vi "LB_AssertIndexValue_Tests.vi"(11 "error in":errorcluster) -> (15 "error out":errorcluster)   [LabVIEW 2016, in "DronaTest.lvlib"]
uses:
  DronaTest.lvlib
  APIs/Stimulus/ControlValue/SetValueAuto.vi
  APIs/Assert/AssertControlValue/Controls/Listbox/AssertIndexValue.vi
  <vilib>/addons/_JKI Toolkits/Caraya/classes/Assert/Assert Error.vi
  <vilib>/addons/_JKI Toolkits/Caraya/classes/Assert/Assert Equal Value_Variant.vi
  <vilib>/addons/_JKI Toolkits/Caraya/classes/Test/Test.lvclass
  Drona.lvlib
  <vilib>/SLL Toolkit/SLL Debug/SLL Debug.lvlib
  <vilib>/addons/_JKI Toolkits/Caraya/classes/Assert/Assert.lvclass
  APIs/Assert/AssertControlValue/Controls/Listbox/AssertListbox.lvlib
  APIs/Stimulus/ControlValue/ControlValue.lvlib
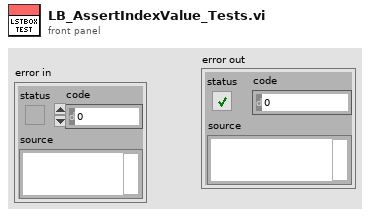
[diagram p1: front panel]
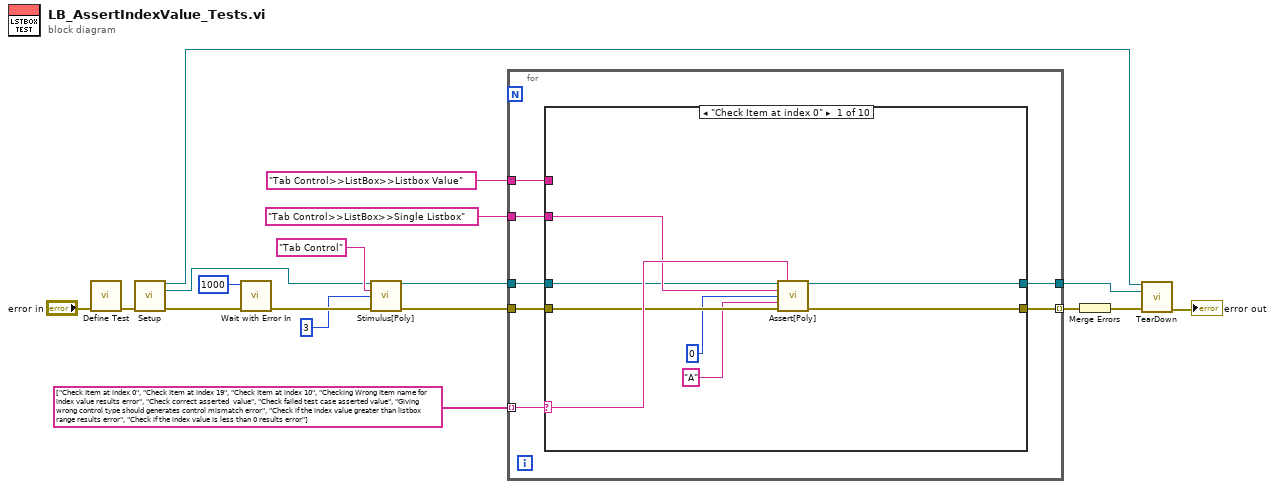
[diagram p0: block diagram]
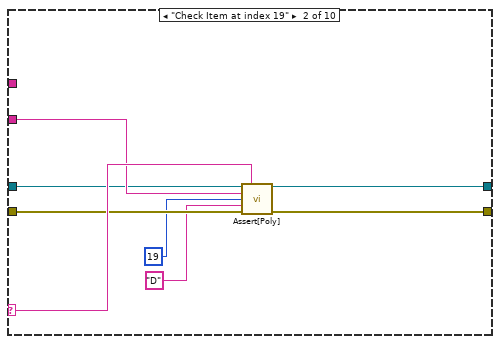
[diagram p2: hidden frame]
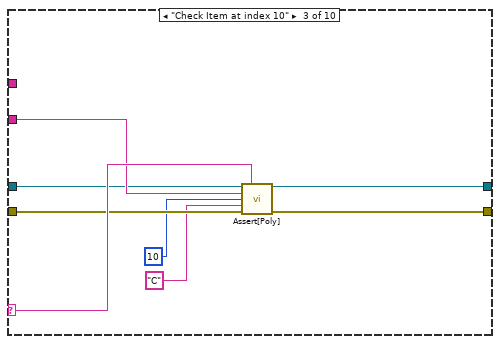
[diagram p3: hidden frame]
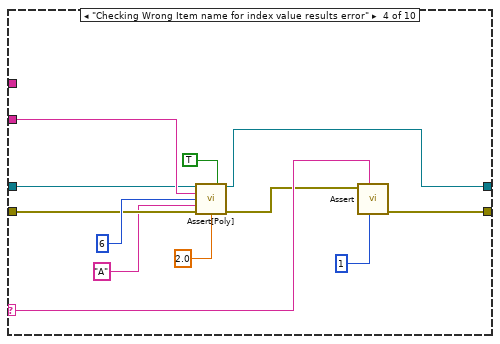
[diagram p4: hidden frame]
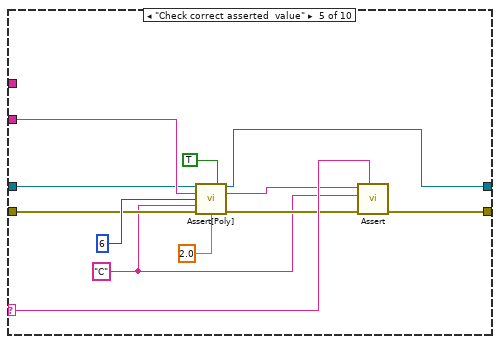
[diagram p5: hidden frame]
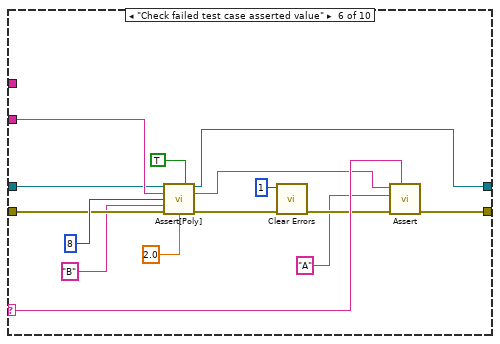
[diagram p6: hidden frame]
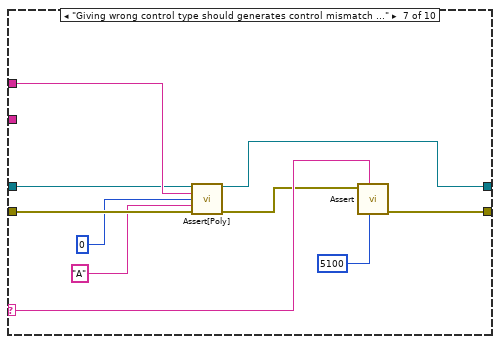
[diagram p7: hidden frame]
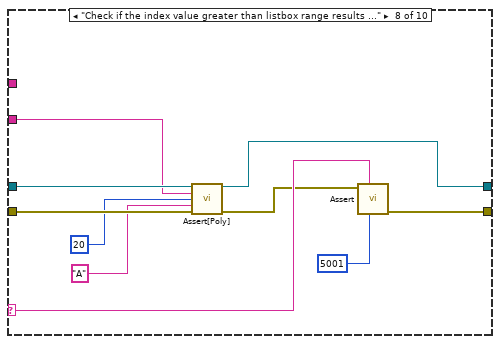
[diagram p8: hidden frame]
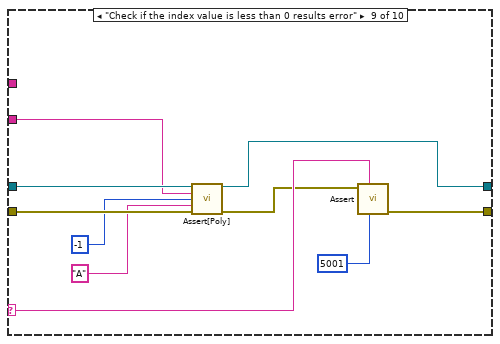
[diagram p9: hidden frame]
diagram:
  n1 = call <vilib>:"Define Test.vi"("error in (no error)"="error in") -> ("error out"=w7:errorcluster)  [unwired: 10 in]
  n2 = call "Setup.vi"("error in (no error)"=w7) -> ("Application Ref"=w3:refnum<vi>, "VI out"=w5:refnum<vi>, "error out"=w6:errorcluster)  [unwired: 12 in]
  n3 = call <vilib>:"Wait with Error In.vi"("error in (no error)"=w6, "milliseconds to wait"=u32 1000) -> ("error out"=w16:errorcluster)  [unwired: 9 in]
  n4 = call-poly "Stimulus[Poly].vi"("VI Reference In"=w5, "Control Path"="Tab Control", "Value (Signaling)"=3, "error in"=w16) -> ("VI Reference Out"=w12:refnum<vi>, "error out"=w15:errorcluster)  [unwired: 10 in]
  n5 = for {
    tunnel: w12 -> [w24]
    tunnel: "Tab Control>>ListBox>>Single Listbox" ("Control Path") -> [w23]
    tunnel: "Tab Control>>ListBox>>Listbox Value" ("Control Path") -> [w22]
    tunnel: string[] ["Check Item at index 0", "Check Item at index 19", "Check Item at index 10", "Checking Wrong Item name for index value results error", "Check correct asserted  value", "Check failed test case asserted value", "Giving wrong control type should generates control mismatch error", "Check if the index value greater than listbox range results error", "Check if the index value is less than 0 results error"] -> [w20] mode=indexing
    tunnel: [w19] -> w2
    tunnel: w15 -> [w25]
    tunnel: [w21] -> w8 mode=indexing
    n6 = case shown="\"Check Item at index 0\"" w20 {
      selector: w20 -> [w31 w39 w47 w60 w72 w87 w97 w107 w117 _]
      tunnel: w25 -> [w29 w37 w45 w52 w67 w82 w92 w103 w113 w120]
      tunnel: w24 -> [w28 w36 w44 w51 w66 w81 w91 w102 w112 w119]
      tunnel: w23 -> [w30 w38 w46 w58 w71 w86 _ w99 w109 _]
      tunnel: w22 -> [_ _ _ _ _ _ w94 _ _ _]
      tunnel: [w33 w41 w49 w61 w73 w88 w98 w108 w118 w120] -> w21
      tunnel: [w32 w40 w48 w56 w69 w84 w93 w104 w114 w119] -> w19
      frame "Check Item at index 0" {
        n7 = call-poly "Assert[Poly].vi"("VI Reference In"=w28, "Test Label"=w31, "Control Path"=w30, "Item Index"=0, "Item Value"="A", "Error In"=w29) -> ("VI Reference Out"=w32:refnum<vi>, "Error Out"=w33:errorcluster)  [unwired: 7 in, 1 out]
      }
      frame "Check Item at index 19" {
        n8 = call-poly "Assert[Poly].vi"("VI Reference In"=w36, "Test Label"=w39, "Control Path"=w38, "Item Index"=19, "Item Value"="D", "Error In"=w37) -> ("VI Reference Out"=w40:refnum<vi>, "Error Out"=w41:errorcluster)  [unwired: 7 in, 1 out]
      }
      frame "Check Item at index 10" {
        n9 = call-poly "Assert[Poly].vi"("VI Reference In"=w44, "Test Label"=w47, "Control Path"=w46, "Item Index"=10, "Item Value"="C", "Error In"=w45) -> ("VI Reference Out"=w48:refnum<vi>, "Error Out"=w49:errorcluster)  [unwired: 7 in, 1 out]
      }
      frame "Checking Wrong Item name for index value results error" {
        n10 = call-poly "Assert[Poly].vi"("VI Reference In"=w51, "Assert Only? (F)"=TRUE, "Control Path"=w58, "Item Index"=6, "Item Value"="A", "Error In"=w52, "Timeout(5 sec)"=2.0) -> ("VI Reference Out"=w56:refnum<vi>, "Error Out"=w55:errorcluster)  [unwired: 6 in, 1 out]
        n11 = call-poly <vilib>:"Assert.vi"("error code (1)"=1, "Label"=w60, "Error?"=w55) -> ("error out"=w61:errorcluster)  [unwired: 8 in]
      }
      frame "Check correct asserted  value" {
        w63 = "C" ("Item Value")
        n12 = call-poly "Assert[Poly].vi"("VI Reference In"=w66, "Assert Only? (F)"=TRUE, "Control Path"=w71, "Item Index"=6, "Item Value"=w63, "Error In"=w67, "Timeout(5 sec)"=2.0) -> ("VI Reference Out"=w69:refnum<vi>, "Asserted Value"=w64:string, "Error Out"=w65:errorcluster)  [unwired: 6 in]
        n13 = call-poly <vilib>:"Assert.vi"("Label"=w72, "error in (no error)"=w65, "Y"=w63, "X"=w64) -> ("error out"=w73:errorcluster)  [unwired: 7 in]
      }
      frame "Check failed test case asserted value" {
        n14 = call-poly "Assert[Poly].vi"("VI Reference In"=w81, "Assert Only? (F)"=TRUE, "Control Path"=w86, "Item Index"=8, "Item Value"="B", "Error In"=w82, "Timeout(5 sec)"=2.0) -> ("VI Reference Out"=w84:refnum<vi>, "Asserted Value"=w79:string, "Error Out"=w80:errorcluster)  [unwired: 6 in]
        n15 = call <vilib>:"Clear Errors.vi"("error in (no error)"=w80, "specific error code to clear (0: all)"=1) -> ("error out"=w77:errorcluster)  [unwired: 4 in, 1 out]
        n16 = call-poly <vilib>:"Assert.vi"("Label"=w87, "error in (no error)"=w77, "Y"="A" ("Item Value"), "X"=w79) -> ("error out"=w88:errorcluster)  [unwired: 7 in]
      }
      frame "Giving wrong control type should generates control mismatch error" {
        n17 = call-poly "Assert[Poly].vi"("VI Reference In"=w91, "Control Path"=w94, "Item Index"=0, "Item Value"="A", "Error In"=w92) -> ("VI Reference Out"=w93:refnum<vi>, "Error Out"=w95:errorcluster)  [unwired: 8 in, 1 out]
        n18 = call-poly <vilib>:"Assert.vi"("error code (1)"=5100, "Label"=w97, "Error?"=w95) -> ("error out"=w98:errorcluster)  [unwired: 8 in]
      }
      frame "Check if the index value greater than listbox range results error" {
        n19 = call-poly "Assert[Poly].vi"("VI Reference In"=w102, "Control Path"=w99, "Item Index"=20, "Item Value"="A", "Error In"=w103) -> ("VI Reference Out"=w104:refnum<vi>, "Error Out"=w105:errorcluster)  [unwired: 8 in, 1 out]
        n20 = call-poly <vilib>:"Assert.vi"("error code (1)"=5001, "Label"=w107, "Error?"=w105) -> ("error out"=w108:errorcluster)  [unwired: 8 in]
      }
      frame "Check if the index value is less than 0 results error" {
        n21 = call-poly "Assert[Poly].vi"("VI Reference In"=w112, "Control Path"=w109, "Item Index"=-1, "Item Value"="A", "Error In"=w113) -> ("VI Reference Out"=w114:refnum<vi>, "Error Out"=w115:errorcluster)  [unwired: 8 in, 1 out]
        n22 = call-poly <vilib>:"Assert.vi"("error code (1)"=5001, "Label"=w117, "Error?"=w115) -> ("error out"=w118:errorcluster)  [unwired: 8 in]
      }
      frame Default {
      }
    }
  }
  n23 = Merge Errors(w8) -> (w4:errorcluster)
  n24 = call "TearDown.vi"("Application Ref"=w3, "VI in"=w2, "error in (no error)"=w4) -> ("error out"=→"error out":errorcluster)  [unwired: 12 in]
